vi "Swerve Rotation Math.vi"(9 "Wheel Speed":dbl, 10 "Wheel Angle":dbl, 11 "Encoder":dbl) -> (2 "Wheel Speed":dbl, 3 "Goal":dbl)   [LabVIEW 2023]
panel:
  # "Goal Angle"
  # "Input"
  # "Current Angle"
  # "in Encoder"
  # "Output"
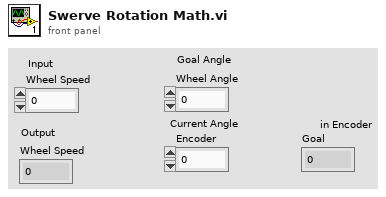
[diagram p1: front panel]
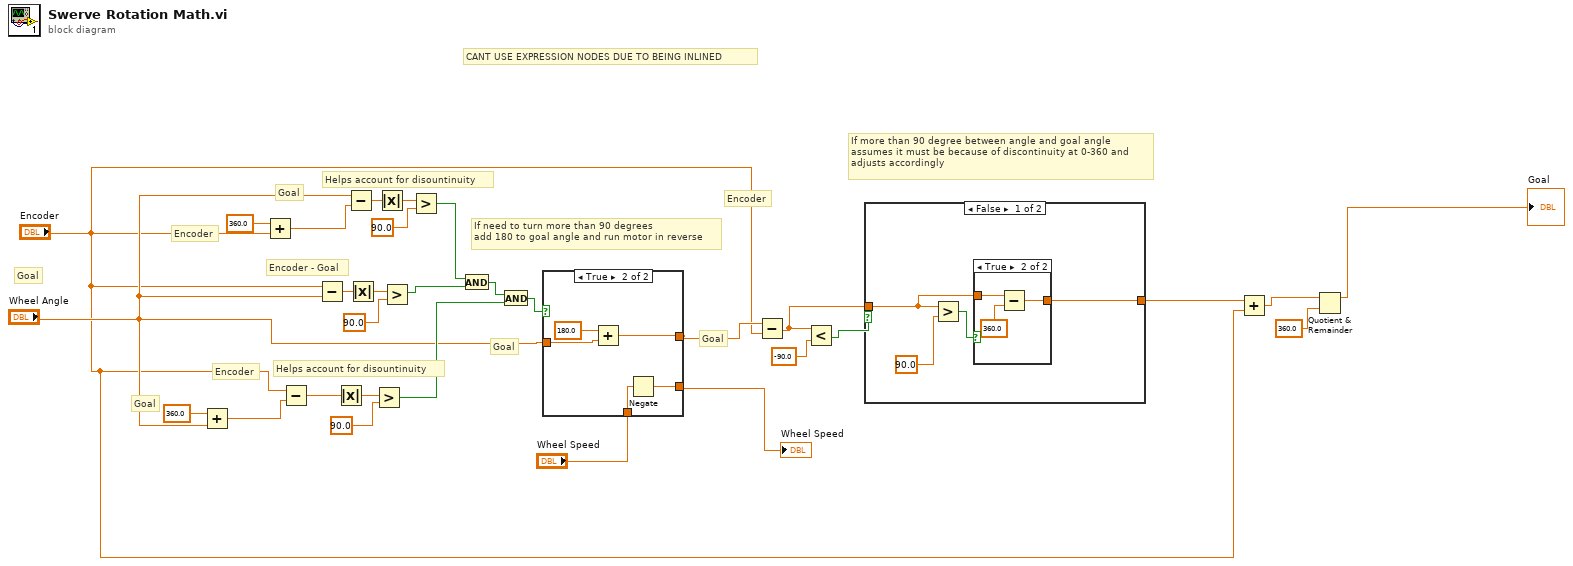
[diagram p0: block diagram]
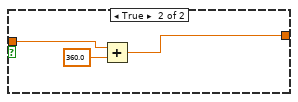
[diagram p3: hidden frame]
diagram:
  # "CANT USE EXPRESSION NODES DUE TO BEING INLINED"
  # "Helps account for disountinuity"
  # "Helps account for disountinuity"
  # "Encoder"
  # "Goal"
  # "Goal"
  # "Goal"
  # "Encoder"
  # "Goal"
  # "Goal"
  # "Encoder"
  # "Encoder - Goal"
  # "If more than 90 degree between angle and goal angle\nassumes it must be because of discontinuity at 0-360 and\nadjusts accordingly"
  # "If need to turn more than 90 degrees\nadd 180 to goal angle and run motor in reverse"
  n1 = Add(x=360.0, y="Wheel Angle") -> (x+y=w8:dbl)
  n2 = Add(x=360.0, y="Encoder") -> (x+y=w11:dbl)
  n3 = Subtract(x="Encoder", y=w8) -> (x-y=w29:dbl)
  n4 = Subtract(x="Encoder", y="Wheel Angle") -> (x-y=w24:dbl)
  n5 = Absolute Value(x=w29) -> (abs(x)=w28:dbl)
  n6 = Subtract(x="Wheel Angle", y=w11) -> (x-y=w30:dbl)
  n7 = Absolute Value(x=w24) -> (abs(x)=w23:dbl)
  n8 = Greater?(x=w28, y=90.0) -> (0:w20:bool)
  n9 = Absolute Value(x=w30) -> (abs(x)=w26:dbl)
  n10 = Greater?(x=w23, y=90.0) -> (0:w18:bool)
  n11 = Greater?(x=w26, y=90.0) -> (0:w17:bool)
  n12 = And(x=w17, y=w18) -> (x .and. y?=w19:bool)
  n13 = And(x=w19, y=w20) -> (x .and. y?=w21:bool)
  n14 = case shown="True" w21 {
    tunnel: "Wheel Angle" -> [w32 w37]
    tunnel: [w32 w35] -> w16
    tunnel: "Wheel Speed" -> [w31 w34]
    tunnel: [w31 w33] -> w9
    frame False {
    }
    frame True {
      n15 = Add(x=180.0, y=w37) -> (x+y=w35:dbl)
      n16 = Negate(x=w34) -> (-x=w33:dbl)
    }
  }
  "Wheel Speed" <- w9
  n17 = Subtract(x=w16, y="Encoder") -> (x-y=w13:dbl)
  n18 = Less?(x=w13, y=-90.0) -> (x < y?=w14:bool)
  n19 = case shown="False" w14 {
    tunnel: [w38 w47] -> w12
    tunnel: w13 -> [w39 w46]
    frame False {
      n20 = Greater?(x=w39, y=90.0) -> (0:w40:bool)
      n21 = case shown="True" w40 {
        tunnel: w39 -> [w42 w45]
        tunnel: [w42 w44] -> w38
        frame False {
        }
        frame True {
          n22 = Subtract(x=w45, y=360.0) -> (x-y=w44:dbl)
        }
      }
    }
    frame True {
      n23 = Add(x=w46, y=360.0) -> (x+y=w47:dbl)
    }
  }
  n24 = Add(x=w12, y="Encoder") -> (x+y=w1:dbl)
  n25 = Quotient & Remainder(x=w1, y=360.0) -> (x-y*floor(x/y)=→"Goal":dbl)  [unwired: 1 out]
